vi "Read NumberOfRobots.vi"(8 "error in (no error)":errorcluster, 11 "FreeBallPlayVSS in":refnum<class "FreeBallPlayVSS.lvclass">) -> (0 "error out":errorcluster, 2 "NumberOfRobots":dbl, 3 "FreeBallPlayVSS out":refnum<class "FreeBallPlayVSS.lvclass">)   [LabVIEW 2020, in "FreeBallPlayVSS.lvclass"]
uses:
  FreeBallPlayVSS.lvclass
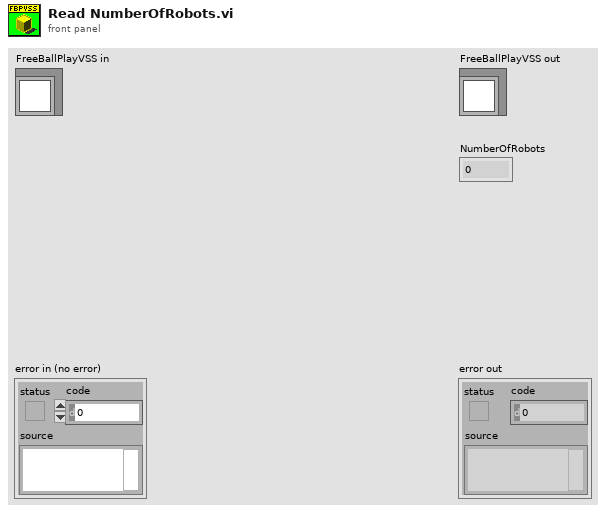
[diagram p1: front panel]
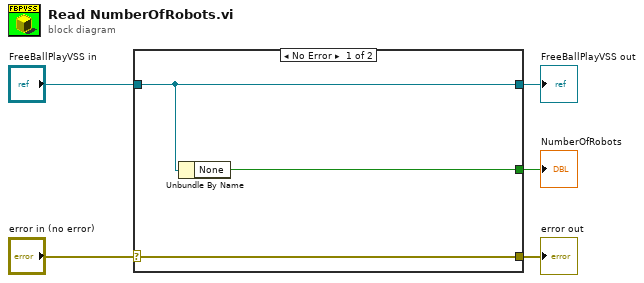
[diagram p0: block diagram]
diagram:
  n1 = case shown="No Error" "error in (no error)" {
    selector: "error in (no error)" -> [w8 w9]
    tunnel: [w8 w9] -> w4
    tunnel: [w7 w10] -> w2
    tunnel: "FreeBallPlayVSS in" -> [w7 w10]
    tunnel: [w6 _] -> w1
    frame No Error {
      n2 = Unbundle By Name(w7) -> ("None"=w6:bool)
    }
    frame Error {
    }
  }
  "error out" <- w4
  "FreeBallPlayVSS out" <- w2
  "NumberOfRobots" <- w1
